vi "createMOT.vi"(8 "error in (no error)":errorcluster, 11 "StaticOutputEditor in":refnum<class "StaticOutputEditor.lvclass">) -> (0 "error out":errorcluster, 3 "StaticOutputEditor out":refnum<class "StaticOutputEditor.lvclass">)   [LabVIEW 2009, in "Views.lvlib" / "ScriptEditor.lvlib" / "StaticOutputEditor.lvclass"]
uses:
  StaticOutputEditor.lvclass
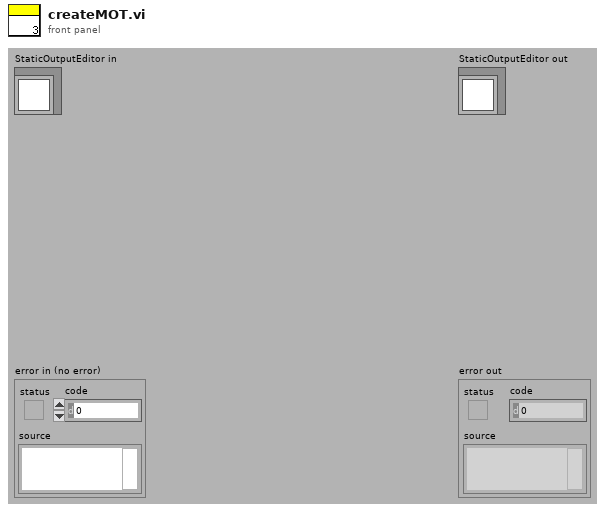
[diagram p1: front panel]
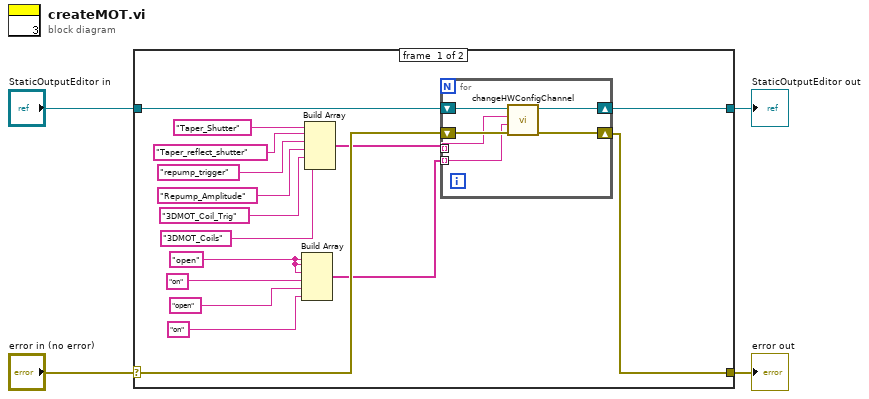
[diagram p0: block diagram]
diagram:
  n1 = case shown="No Error" "error in (no error)" {
    selector: "error in (no error)" -> [w18 w28]
    tunnel: [w17 w28] -> w3
    tunnel: [w19 w27] -> w1
    tunnel: "StaticOutputEditor in" -> [w20 w27]
    frame #0 {
      w5 = "open"
      n2 = Build Array(w5, w5, w5, "on", "open", "on") -> (w12:string[])
      n3 = Build Array("Taper_Shutter", "Taper_reflect_shutter", "repump_trigger", "Repump_Amplitude", "3DMOT_Coil_Trig", "3DMOT_Coils") -> (w15:string[])
      n4 = for {
        shift-right: [w23] -> w17
        shift-left: w18 -> [w24]
        shift-right: [w25] -> w19
        shift-left: w20 -> [w26]
        tunnel: w15 -> [w22] mode=indexing
        tunnel: w12 -> [w21] mode=indexing
        n5 = call "changeHWConfigChannel.vi"("error in (no error)"=w24, "state"=w21, "channel"=w22, "StaticOutputEditor in"=w26) -> ("error out"=w23:errorcluster, "StaticOutputEditor out"=w25:refnum<class "StaticOutputEditor.lvclass">)  [unwired: 6 in]
      }
    }
    frame #1 {
    }
  }
  "error out" <- w3
  "StaticOutputEditor out" <- w1
